vi "Put RT INI.vi"(8 "error in (no error)":errorcluster, 10 "Local RT INI path":path, 11 "RT Management in":refnum<class "RT Management.lvclass">) -> (0 "error out":errorcluster, 3 "RT Management out":refnum<class "RT Management.lvclass">)   [LabVIEW 2015, in "RT Management.lvlib" / "RT Management.lvclass"]
doc: "Puts a local RT INI file onto the target. The default location for PharLap and VxWorks targets is \"ni-rt.ini\" and for Linux targets is \"etc/natinst/share/ni-rt.ini\"."
uses:
  RT Management.lvclass
  File Transfer Behavior/File Transfer Behavior.lvclass
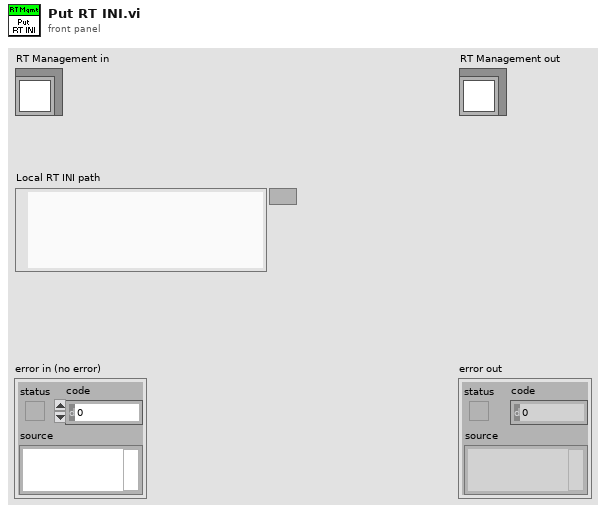
[diagram p1: front panel]
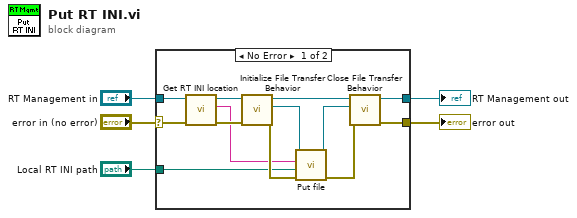
[diagram p0: block diagram]
diagram:
  n1 = case shown="No Error" "error in (no error)" {
    selector: "error in (no error)" -> [w17 w20]
    tunnel: [w8 w20] -> w2
    tunnel: [w10 w19] -> w3
    tunnel: "RT Management in" -> [w16 w19]
    tunnel: "Local RT INI path" -> [w15 _]
    frame No Error {
      n2 = call "Get RT INI location.vi"("error in (no error)"=w17, "RT Management in"=w16) -> ("error out"=w7:errorcluster, "RT INI Location"=w6:string, "RT Management out"=w14:refnum<class "RT Management.lvclass">)  [unwired: 7 in]
      n3 = call "Initialize File Transfer Behavior.vi"("error in (no error)"=w7, "RT Management in"=w14) -> ("error out"=w18:errorcluster, "File Transfer Behavior out"=w13:refnum<class "File Transfer Behavior.lvclass">, "RT Management out"=w12:refnum<class "RT Management.lvclass">)  [unwired: 7 in]
      n4 = call-dynamic "Put file.vi"("error in (no error)"=w18, "Local path"=w15, "Remote path"=w6, "File Transfer Behavior in"=w13) -> ("error out"=w9:errorcluster, "File Transfer Behavior out"=w11:refnum<class "File Transfer Behavior.lvclass">)  [unwired: 6 in]
      n5 = call "Close File Transfer Behavior.vi"("error in (no error)"=w9, "File Transfer Behavior in"=w11, "RT Management in"=w12) -> ("error out"=w8:errorcluster, "RT Management out"=w10:refnum<class "RT Management.lvclass">)  [unwired: 7 in]
    }
    frame Error {
    }
  }
  "error out" <- w2
  "RT Management out" <- w3
